vi "ComputerRemoteForOldJoystick.vi"() -> ()   [LabVIEW 2020]
uses:
  oldStudicaJoystick.ctl
  <vilib>/Utility/inputDevices.llb/joystickAcquire.vi
  <vilib>/Utility/inputDevices.llb/closeJoystick.vi
  <vilib>/ReMiSYS Technology/RemoteToolkit/Sender/Sender.lvclass
panel:
  out "StudicaJoystick":T1
  in  "IP Address":string="10.12.34.2"
  in  "Stop Button":bool
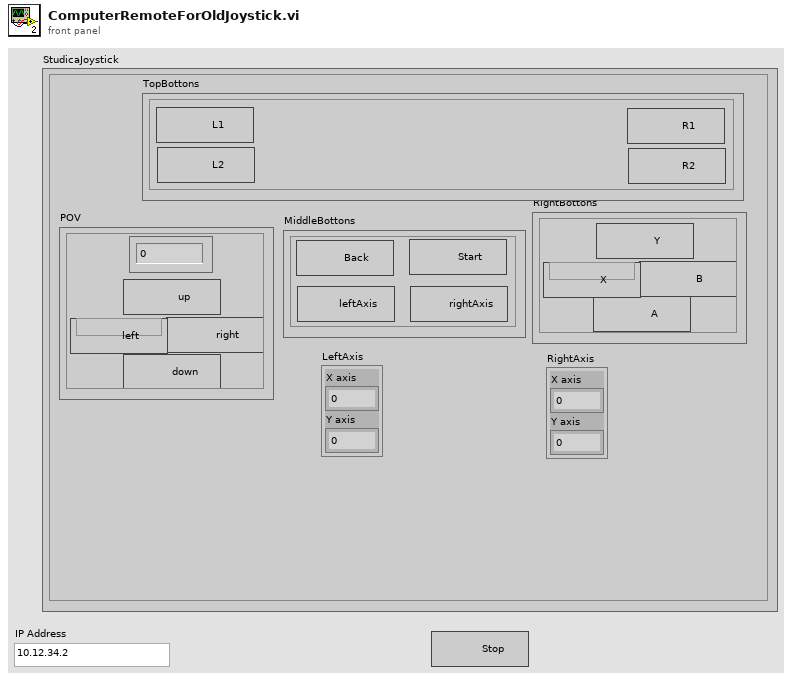
[diagram p1: front panel]
types:
  T1 = typedef "oldStudicaJoystick.ctl" = cluster{"LeftAxis":cluster{"X axis":i32, "Y axis":i32}, "RightAxis":cluster{"X axis":i32, "Y axis":i32}, "RightBottons":cluster{"A":bool, "B":bool, "X":bool, "Y":bool}, "TopBottons":cluster{"Left1":bool, "Left2":bool, "Right1":bool, "Right2":bool}, "MiddleBottons":cluster{"Back":bool, "Play Button":bool, "leftAxis":bool, "rightAxis":bool}, "POV":cluster{"right":bool, "left":bool, "up":bool, "direction":i32, "down":bool}}
  T2 = cluster{"X axis":i32, "Y axis":i32, "Z axis":i32, "X axis rotation":i32, "Y axis rotation":i32, "Z axis rotation":i32, "U axis":i32, "V axis":i32}
  T3 = cluster{"button 1":bool, "button 2":bool, "button 3":bool, "button 4":bool, "button 5":bool, "button 6":bool, "button 7":bool, "button 8":bool, "button 9":bool, "button 10":bool, "button 11":bool, "button 12":bool, "button 13":bool, "button 14":bool, "button 15":bool, "button 16":bool, "button 17":bool, "button 18":bool, "button 19":bool, "button 20":bool, "button 21":bool, "button 22":bool, "button 23":bool, "button 24":bool, "button 25":bool, "button 26":bool, "button 27":bool, "button 28":bool, "button 29":bool, "button 30":bool, "button 31":bool, "button 32":bool}
  T4 = cluster{"pov 1":i32, "pov 2":i32, "pov 3":i32, "pov 4":i32}
  T5 = cluster{"X axis rotation":i32, "Y axis rotation":i32}
  T6 = cluster{"button 5":bool, bool, "button 6":bool, bool}
  T7 = cluster{"button 1":bool, "button 2":bool, "button 3":bool, "button 4":bool}
  T8 = cluster{"button 7":bool, "button 8":bool, "button 9":bool, "button 10":bool}
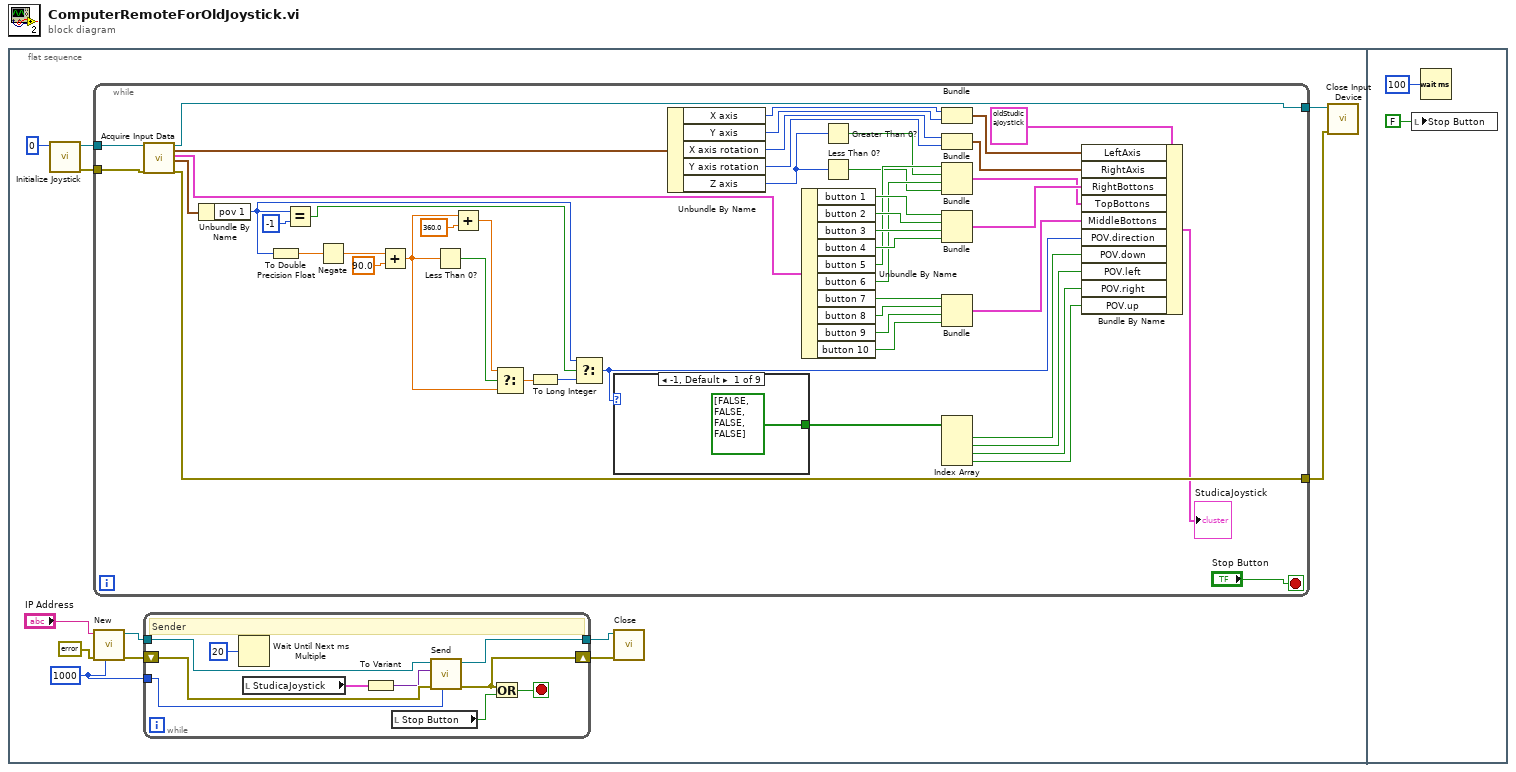
[diagram p0: block diagram]
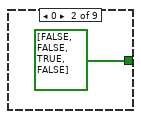
[diagram p2: hidden frame]
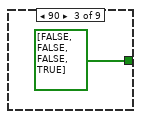
[diagram p3: hidden frame]
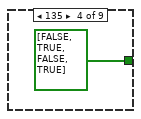
[diagram p4: hidden frame]
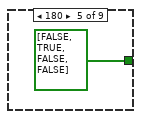
[diagram p5: hidden frame]
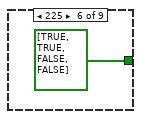
[diagram p6: hidden frame]
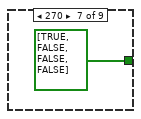
[diagram p7: hidden frame]
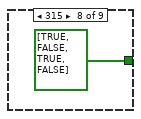
[diagram p8: hidden frame]
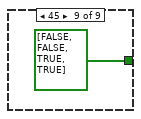
[diagram p9: hidden frame]
diagram:
  n1 = flat-sequence {
    frame #0 {
      w5 = 1000 ("Timeout ms (25000)")
      n2 = call <vilib>:"Initialize Joystick.vi"("device index"=0) -> ("error out"=w12:errorcluster, "device ID"=w9:refnum<k1>)  [unwired: 9 in]
      n3 = while {
        tunnel: w12 -> [w71]
        tunnel: [w70] -> w11
        tunnel: w9 -> [w69]
        tunnel: [w68] -> w8
        stop <- "Stop Button" stop-if-true
        n4 = call-poly <vilib>:"Acquire Input Data.vi"("device ID"=w69, "error in (no error)"=w71) -> ("device ID"=w68:refnum<k1>, "axis info"=w67:T2, "button info"=w59:T3, "direction info"=w42:T4, "error out"=w70:errorcluster)  [unwired: 13 in]
        n5 = Unbundle By Name(w42) -> ("pov 1"=w25:i32)
        n6 = To Double Precision Float(number=w25) -> (double precision float=w41:dbl)
        n7 = Equal?(x=w25, y=-1) -> (x = y?=w27:bool)
        n8 = Negate(x=w41) -> (-x=w40:dbl)
        n9 = Add(x=w40, y=90.0) -> (x+y=w30:dbl)
        n10 = Less Than 0?(x=w30) -> (x < 0?=w32:bool)
        n11 = Add(x=w30, y=360.0) -> (x+y=w31:dbl)
        n12 = Select(t=w31, s=w32, f=w30) -> (s? t:f=w29:dbl)
        n13 = To Long Integer(number=w29) -> (32bit integer=w24:i32)
        n14 = Select(t=w25, s=w27, f=w24) -> (s? t:f=w26:i32)
        n15 = case shown="-1, Default" w26 {
          tunnel: [bool[] [FALSE, FALSE, FALSE, FALSE] bool[] [FALSE, FALSE, TRUE, FALSE] bool[] [FALSE, FALSE, FALSE, TRUE] bool[] [FALSE, TRUE, FALSE, TRUE] bool[] [FALSE, TRUE, FALSE, FALSE] bool[] [TRUE, TRUE, FALSE, FALSE] bool[] [TRUE, FALSE, FALSE, FALSE] bool[] [TRUE, FALSE, TRUE, FALSE] bool[] [FALSE, FALSE, TRUE, TRUE]] -> w38
          frame -1, Default {
          }
          frame 0 {
          }
          frame 90 {
          }
          frame 135 {
          }
          frame 180 {
          }
          frame 225 {
          }
          frame 270 {
          }
          frame 315 {
          }
          frame 45 {
          }
        }
        n16 = Unbundle By Name(w67) -> ("X axis"=w66:i32, "Y axis"=w65:i32, "X axis rotation"=w63:i32, "Y axis rotation"=w62:i32, "Z axis"=w50:i32)
        n17 = Unbundle By Name(w59) -> ("button 1"=w58:bool, "button 2"=w57:bool, "button 3"=w56:bool, "button 4"=w55:bool, "button 5"=w53:bool, "button 6"=w52:bool, "button 7"=w47:bool, "button 8"=w46:bool, "button 9"=w45:bool, "button 10"=w44:bool)
        n18 = Greater Than 0?(x=w50) -> (x > 0?=w51:bool)
        n19 = Less Than 0?(x=w50) -> (x < 0?=w49:bool)
        n20 = Bundle("X axis"=w66, "Y axis"=w65) -> (w64:cluster{"X axis":i32, "Y axis":i32})  [unwired: 1 in]
        n21 = Bundle("X axis rotation"=w63, "Y axis rotation"=w62) -> (w61:T5)  [unwired: 1 in]
        n22 = Bundle("button 5"=w53, w51, "button 6"=w52, w49) -> (w48:T6)  [unwired: 1 in]
        n23 = Bundle("button 1"=w58, "button 2"=w57, "button 3"=w56, "button 4"=w55) -> (w54:T7)  [unwired: 1 in]
        n24 = Bundle("button 7"=w47, "button 8"=w46, "button 9"=w45, "button 10"=w44) -> (w43:T8)  [unwired: 1 in]
        n25 = Index Array(array=w38) -> (element #1=w37:bool, element #2=w36:bool, element #3=w35:bool, element #4=w34:bool)  [unwired: 4 in]
        n26 = Bundle By Name(cluster=T1 {"LeftAxis"={"X axis"=0, "Y axis"=0}, "RightAxis"={"X axis"=0, "Y axis"=0}, "RightBottons"={"A"=FALSE, "B"=FALSE, "X"=FALSE, "Y"=FALSE}, "TopBottons"={"Left1"=FALSE, "Left2"=FALSE, "Right1"=FALSE, "Right2"=FALSE}, "MiddleBottons"={"Back"=FALSE, "Play Button"=FALSE, "leftAxis"=FALSE, "rightAxis"=FALSE}, "POV"={"right"=FALSE, "left"=FALSE, "up"=FALSE, "direction"=0, "down"=FALSE}} ("OldStudicaJoystick"), "LeftAxis"=w64, "RightAxis"=w61, "RightBottons"=w54, "TopBottons"=w48, "MiddleBottons"=w43, "POV.direction"=w26, "POV.down"=w37, "POV.left"=w36, "POV.right"=w35, "POV.up"=w34) -> (→"StudicaJoystick":T1)
      }
      n27 = call <vilib>:"New.vi"("Timeout ms (25000)"=w5, "Error In"=errorcluster {"status"=FALSE, "code"=0, "source"=""}, "IP Address"="IP Address") -> ("Error Out"=w6:errorcluster, "Sender Ref."=w3:refnum<class "Sender.lvclass">)  [unwired: 7 in]
      n28 = while {
        shift-right: [w18] -> w2
        shift-left: w6 -> [w20]
        tunnel: w3 -> [w21]
        tunnel: w5 -> [w16]
        tunnel: [w19] -> w1
        stop <- w22 stop-if-true
        # "Sender"
        n29 = Wait Until Next ms Multiple(millisecond multiple=u32 20) -> ()  [unwired: 1 out]
        n30 = local read "StudicaJoystick"() -> (w13:T1)
        n31 = To Variant(anything=w13) -> (Variant=w17:variant)
        n32 = local read "Stop Button"() -> (w14:bool)
        n33 = call <vilib>:"Send.vi"("Timeout ms (1000)"=w16, "Error In"=w20, "Value"=w17, "Sender Ref."=w21) -> ("Error Out"=w18:errorcluster, "Sender Ref."=w19:refnum<class "Sender.lvclass">)  [unwired: 6 in]
        n34 = Or(x=w18, y=w14) -> (x .or. y?=w22:bool)
      }
      n35 = call <vilib>:"Close.vi"("Error In"=w2, "Receiver Ref."=w1) -> ()  [unwired: 9 in, 1 out]
      n36 = call-poly <vilib>:"Close Input Device.vi"("error in (no error)"=w11, "device ID"=w8) -> ()  [unwired: 8 in, 1 out]
    }
    frame #1 {
      n37 = local write "Stop Button"(FALSE ("Stop Button")) -> ()
      n38 = Wait (ms)(milliseconds to wait=u32 100) -> ()  [unwired: 1 out]
    }
  }
